vi "Write sync us timeout.vi"(8 "error in (no error)":errorcluster, 10 "sync us timeout":i32, 11 "Shared Memory configuration in":refnum<class "Shared Memory configuration.lvclass">) -> (0 "error out":errorcluster, 3 "Shared Memory configuration out":refnum<class "Shared Memory configuration.lvclass">)   [LabVIEW 2013, in "Shared Memory configuration.lvclass"]
uses:
  Shared Memory configuration.lvclass
  Shared Memory configuration.lvclass/Shared Memory configuration.ctl
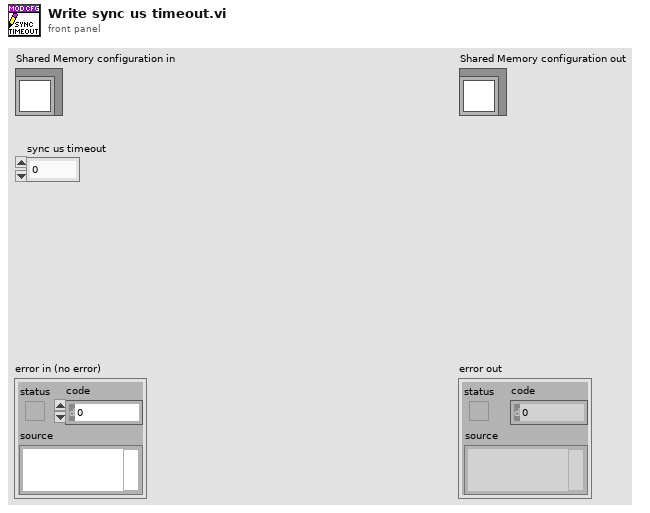
[diagram p1: front panel]
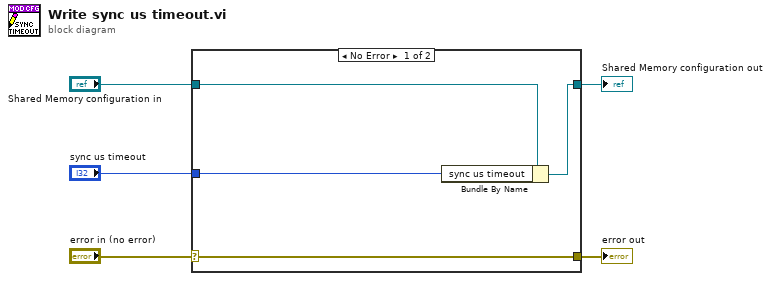
[diagram p0: block diagram]
diagram:
  n1 = case shown="No Error" "error in (no error)" {
    selector: "error in (no error)" -> [w9 w10]
    tunnel: [w9 w10] -> w4
    tunnel: [w7 w11] -> w2
    tunnel: "Shared Memory configuration in" -> [w8 w11]
    tunnel: "sync us timeout" -> [w6 _]
    frame No Error {
      n2 = Bundle By Name(cluster=w8, "sync us timeout"=w6) -> (w7:refnum<class "Shared Memory configuration.lvclass">)
    }
    frame Error {
    }
  }
  "error out" <- w4
  "Shared Memory configuration out" <- w2
